vi "Read Latest Measurement.vi"(8 "error in (no error)":errorcluster, 11 "VISA resource name":refnum<visa-resource-name>) -> (0 "error out":errorcluster, 1 "Measurement Metadata":T1, 2 "Measurement":dbl, 3 "VISA resource name out":refnum<visa-resource-name>)   [LabVIEW 2019, in "Keithley 2182.lvlib"]
doc: "Reads the latest measurement taken by the instrument."
uses:
  Keithley 2182.lvlib
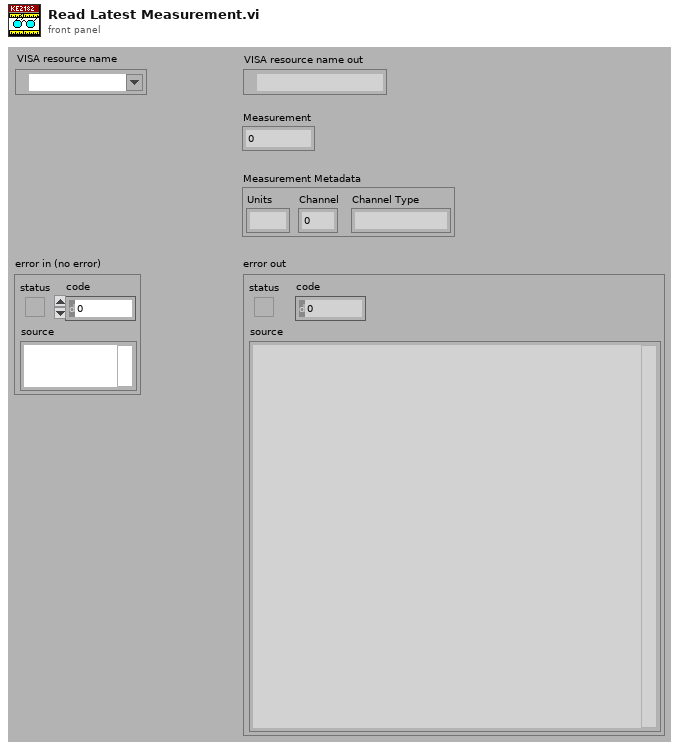
[diagram p1: front panel]
types:
  T1 = cluster{"Units":string, "Channel":i32, "Channel Type":string}
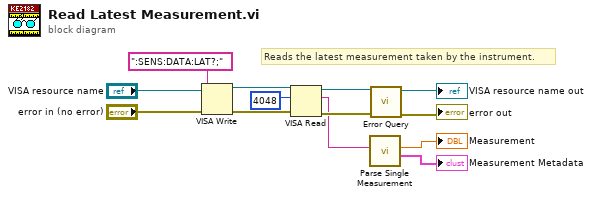
[diagram p0: block diagram]
diagram:
  # "Reads the latest measurement taken by the instrument."
  n1 = VISA Write(VISA resource name="VISA resource name", write buffer=":SENS:DATA:LAT?;", error in (no error)="error in (no error)") -> (VISA resource name out=w9:refnum<visa-resource-name>, error out=w10:errorcluster)  [unwired: 1 out]
  n2 = VISA Read(VISA resource name=w9, byte count=u32 4048, error in (no error)=w10) -> (VISA resource name out=w4:refnum<visa-resource-name>, read buffer=w3:string, error out=w5:errorcluster)  [unwired: 1 out]
  n3 = call "Parse Single Measurement.vi"("Measurement String"=w3) -> ("Measurement Metadata"=→"Measurement Metadata":T1, "Measurement"=→"Measurement":dbl)  [unwired: 8 in, 1 out]
  n4 = call "Error Query.vi"("error in (no error)"=w5, "VISA resource name"=w4) -> ("error out"=→"error out":errorcluster, "VISA resource name out"=→"VISA resource name out":refnum<visa-resource-name>)  [unwired: 6 in, 2 out]
